vi "MCSPmtReadout.vi"() -> (1 "pmtOut":u8)   [LabVIEW 2014]
uses:
  <vilib>/rvi/eio/common/nirviEmuTemplateMethod_errors.vi
  <vilib>/eio/EIONode/EIONode.xnode
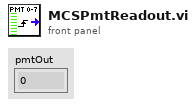
[diagram p1: front panel]
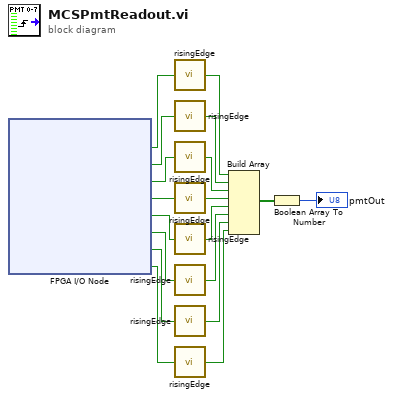
[diagram p0: block diagram]
diagram:
  n1 = xnode "FPGA I/O Node"() -> ("Connector1/DIO16"=w18:bool, "Connector1/DIO17"=w17:bool, "Connector1/DIO18"=w16:bool, "Connector1/DIO19"=w15:bool, "Connector1/DIO20"=w14:bool, "Connector1/DIO21"=w13:bool, "Connector1/DIO22"=w12:bool, "Connector1/DIO23"=w11:bool)  [unwired: 8 in, 8 out]
  n2 = call "risingEdge.vi"("In"=w18) -> ("out"=w10:bool)
  n3 = call "risingEdge.vi"("In"=w17) -> ("out"=w9:bool)
  n4 = call "risingEdge.vi"("In"=w16) -> ("out"=w8:bool)
  n5 = call "risingEdge.vi"("In"=w15) -> ("out"=w7:bool)
  n6 = call "risingEdge.vi"("In"=w14) -> ("out"=w6:bool)
  n7 = call "risingEdge.vi"("In"=w13) -> ("out"=w5:bool)
  n8 = call "risingEdge.vi"("In"=w12) -> ("out"=w4:bool)
  n9 = call "risingEdge.vi"("In"=w11) -> ("out"=w3:bool)
  n10 = Build Array(w10, w9, w8, w7, w6, w5, w4, w3) -> (w2:bool[])
  n11 = Boolean Array To Number(Boolean array=w2) -> (number=→"pmtOut":u8)
